vi "Teleop.vi"(10 "Match Info":T1={"Autonomous Elapsed Seconds"=0.0, "TeleOp Elapsed Seconds"=0.0, "Disabled Elapsed Seconds"=0.0, "Visited Autonomous"=FALSE, "Visited TeleOp"=FALSE, "Visited Disabled"=FALSE, "Autonomous Settings"={"Autonomous Style"=enum."Independent", "VI Refnum"=refnum}}, 11 "Call Context":T2) -> ()   [LabVIEW 2018]
doc: "This VI is called for each TeleOp packet received from the DS where the robot is not disabled. It is often used to read from the joysticks and update I/O or to update setpoints for timed control loops. It should complete and return within 20 milliseconds or it may miss DS packets."
uses:
  <vilib>/Rock Robotics/WPI/DriverStation/WPI_DriverStationDerivedRobotMode.ctl
  <vilib>/Rock Robotics/WPI/DriverStation/WPI_DriverStationMatch Info.ctl
  <vilib>/Rock Robotics/WPI/Utilities/WPI_GetSetVariantRefNum.vi
  Robot Global Data.vi
  Support Code/Valkyrie1Buttons.vi
panel:
  out "LB":bool
  out "RB":bool
  out "<":bool
  out ">":bool
  out "\\/":bool
  out "/\\":bool=TRUE
  out "X":bool
  out "B":bool
  out "A":bool
  out "Y":bool
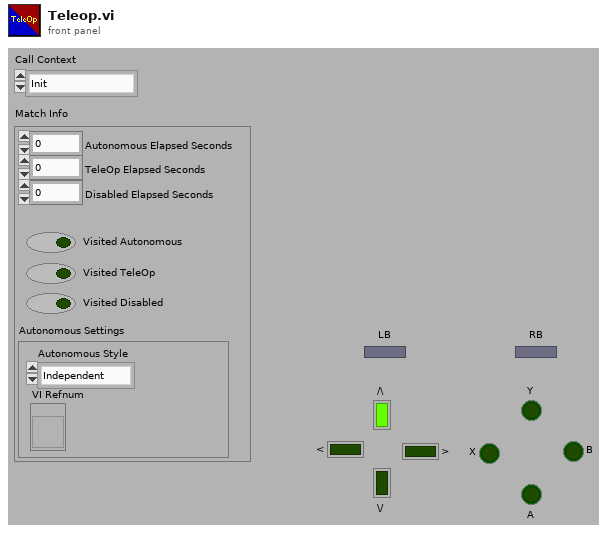
[diagram p1: front panel]
types:
  T1 = typedef "WPI_DriverStationMatch Info.ctl" = cluster{"Autonomous Elapsed Seconds":dbl, "TeleOp Elapsed Seconds":dbl, "Disabled Elapsed Seconds":dbl, "Visited Autonomous":bool, "Visited TeleOp":bool, "Visited Disabled":bool, "Autonomous Settings":cluster{"Autonomous Style":enum16{"Iterative", "Independent"}, "VI Refnum":refnum<vi>}}
  T2 = typedef "WPI_DriverStationDerivedRobotMode.ctl" = enum16{"Init", "Execute", "Stop"}
  T3 = typedef "WPI_JoystickDevRef.ctl" = cluster{"Device":T4}
  T4 = typedef "WPI_JoystickDeviceEnum.ctl" = enum16{"USB 0", "USB 1", "USB 2", "USB 3", "USB 4", "USB 5"}
  T5 = typedef "D-Pad.ctl" = cluster{"Top":bool, "Bottom":bool, "None":bool, "Right":bool, "Left":bool}
  T6 = typedef "Button Cluster.ctl" = cluster{"Buttons[0]":bool, "Buttons[1]":bool, "Buttons[2]":bool, "Buttons[3]":bool, "Buttons[4]":bool, "Buttons[5]":bool, "Buttons[6]":bool, "Buttons[7]":bool, "Buttons[8]":bool, "Buttons[9]":bool}
  T7 = typedef "Axes Cluster.ctl" = cluster{"Axes[0]":dbl, "Axes[1]":dbl, "Axes[2]":dbl, "Axes[3]":dbl, "Axes[4]":dbl, "Axes[5]":dbl, "Axes[6]":dbl, "Axes[7]":dbl, "Axes[8]":dbl}
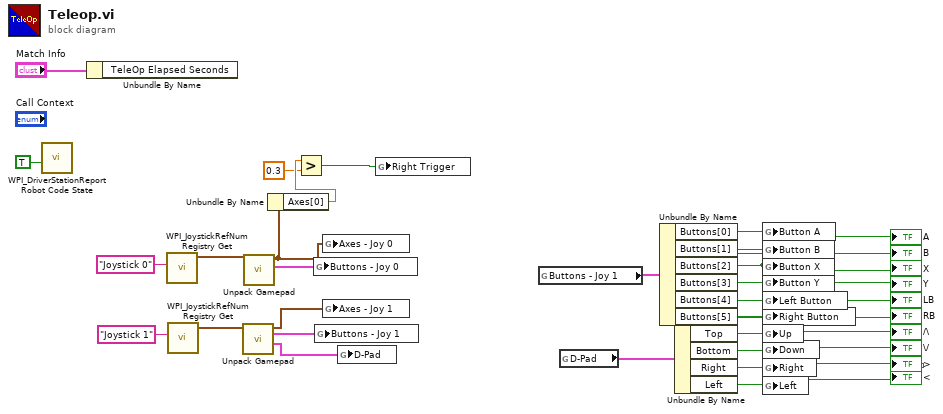
[diagram p0: block diagram]
diagram:
  n1 = call <vilib>:"WPI_DriverStationReport Robot Code State.vi"("TeleOp"=TRUE ("Autonomous")) -> ()  [unwired: 10 in, 1 out]
  n2 = Unbundle By Name("Match Info") -> ()  [unwired: 1 out]
  n3 = call <vilib>:"WPI_JoystickRefNum Registry Get.vi"("refnum name"="Joystick 0") -> ("JoystickDevRef"=w22:T3)  [unwired: 1 in, 9 out]
  n4 = call <vilib>:"WPI_JoystickRefNum Registry Get.vi"("refnum name"="Joystick 1") -> ("JoystickDevRef"=w21:T3)  [unwired: 1 in, 9 out]
  n5 = call "Unpack Gamepad.vi"("JoystickDevRef"=w21) -> ("D-Pad"=w19:T5, "Button Cluster"=w18:T6, "Axes"=w17:T7)  [unwired: 8 in]
  n6 = call "Unpack Gamepad.vi"("JoystickDevRef"=w22) -> ("Button Cluster"=w20:T6, "Axes"=w4:T7)  [unwired: 8 in, 1 out]
  n7 = Unbundle By Name(w4) -> ("Axes[0]"=w3:dbl)
  n8 = Greater?(x=w3, y=0.3) -> (0:w1:bool)
  n9 = global write "Robot Global Data.vi" "Buttons - Joy 0"(w20) -> ()
  n10 = global write "Robot Global Data.vi" "Buttons - Joy 1"(w18) -> ()
  n11 = global write "Robot Global Data.vi" "Axes - Joy 0"(w4) -> ()
  n12 = global write "Robot Global Data.vi" "Axes - Joy 1"(w17) -> ()
  n13 = global write "Robot Global Data.vi" "D-Pad"(w19) -> ()
  n14 = global write "Valkyrie1Buttons.vi" "Right Trigger"(w1) -> ()
  n15 = global read "Robot Global Data.vi" "Buttons - Joy 1"() -> (w16:T6)
  n16 = global read "Robot Global Data.vi" "D-Pad"() -> (w15:T5)
  n17 = Unbundle By Name(w16) -> ("Buttons[0]"=w14:bool, "Buttons[1]"=w13:bool, "Buttons[2]"=w12:bool, "Buttons[3]"=w11:bool, "Buttons[4]"=w5:bool, "Buttons[5]"=w6:bool)
  "Y" <- w11
  "A" <- w14
  "B" <- w13
  "X" <- w12
  "RB" <- w6
  "LB" <- w5
  n18 = Unbundle By Name(w15) -> ("Top"=w7:bool, "Bottom"=w8:bool, "Right"=w9:bool, "Left"=w10:bool)
  "/\\" <- w7
  "\\/" <- w8
  ">" <- w9
  "<" <- w10
  n19 = global write "Valkyrie1Buttons.vi" "Button A"(w14) -> ()
  n20 = global write "Valkyrie1Buttons.vi" "Button B"(w13) -> ()
  n21 = global write "Valkyrie1Buttons.vi" "Button X"(w12) -> ()
  n22 = global write "Valkyrie1Buttons.vi" "Button Y"(w11) -> ()
  n23 = global write "Valkyrie1Buttons.vi" "Left Button"(w5) -> ()
  n24 = global write "Valkyrie1Buttons.vi" "Right Button"(w6) -> ()
  n25 = global write "Valkyrie1Buttons.vi" "Up"(w7) -> ()
  n26 = global write "Valkyrie1Buttons.vi" "Down"(w8) -> ()
  n27 = global write "Valkyrie1Buttons.vi" "Right"(w9) -> ()
  n28 = global write "Valkyrie1Buttons.vi" "Left"(w10) -> ()
